vi "A_New Set Point.vi"(0 "T1":dbl, 1 "T2":dbl, 2 "T3":dbl, 3 "T4":dbl, 4 "T5":dbl, 5 "T6":dbl, 6 "T7":dbl, 8 "T8":dbl, 9 "Period":dbl, 10 "T9":dbl, 11 "i":i32, 12 "T10":dbl, 14 "A1":dbl, 15 "A2":dbl, 16 "A3":dbl, 17 "A4":dbl, 18 "A5":dbl, 19 "A6":dbl) -> (13 "y":dbl)   [LabVIEW 2011]
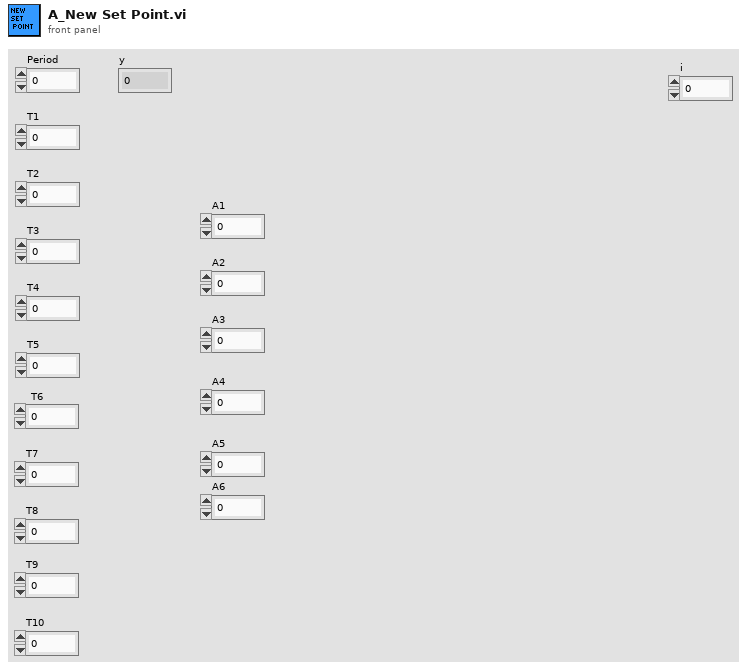
[diagram p1: front panel]
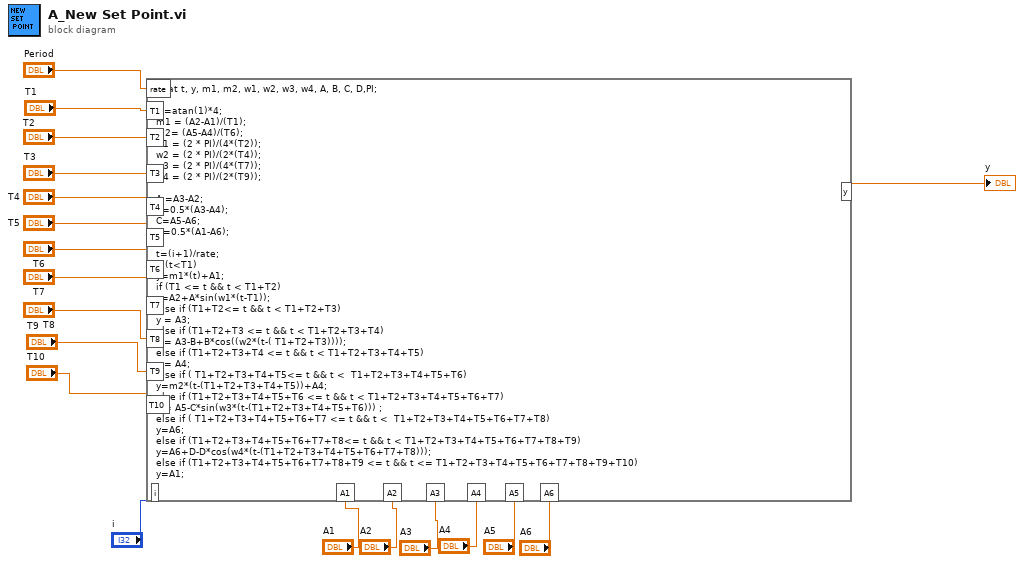
[diagram p0: block diagram]
diagram:
  n1 = formula code="float t, y, m1, m2, w1, w2, w3, w4, A, B, C, D,PI;\n\nPI=atan(1)*4;\nm1 = (A2-A1)/(T1);\nm2= (A5-A4)/(T6);\nw1 = (2 * PI)/(4*(T2));\nw2 = (2 * PI)/(2*(T4));\nw3 = (2 * PI)/(4*(T7));\nw4 = (2 * PI)/(2*(T9));\n\nA =A3-A2;\nB=0.5*(A3-A4);\nC=A5-A6;\nD=0.5*(A1-A6);\n\nt=(i+1)/rate;\nif (t<T1)\ny=m1*(t)+A1;\nif (T1 <= t && t < T1+T2)\ny=A2+A*sin(w1*(t-T1));\nelse if (T1+T2<= t && t < T1+T2+T3)\ny = A3;\nelse if (T1+T2+T3 <= t && t < T1+T2+T3+T4)\ny = A3-B+B*cos((w2*(t-( T1+T2+T3))));\nelse if (T1+T2+T3+T4 <= t && t < T1+T2+T3+T4+T5)\ny = A4;\nelse if ( T1+T2+T3+T4+T5<= t && t <  T1+T2+T3+T4+T5+T6)\ny=m2*(t-(T1+T2+T3+T4+T5))+A4;\nelse if (T1+T2+T3+T4+T5+T6 <= t && t < T1+T2+T3+T4+T5+T6+T7)\ny = A5-C*sin(w3*(t-(T1+T2+T3+T4+T5+T6))) ;\nelse if ( T1+T2+T3+T4+T5+T6+T7 <= t && t <  T1+T2+T3+T4+T5+T6+T7+T8)\ny=A6;\nelse if (T1+T2+T3+T4+T5+T6+T7+T8<= t && t < T1+T2+T3+T4+T5+T6+T7+T8+T9)\ny=A6+D-D*cos(w4*(t-(T1+T2+T3+T4+T5+T6+T7+T8)));\nelse if (T1+T2+T3+T4+T5+T6+T7+T8+T9 <= t && t <= T1+T2+T3+T4+T5+T6+T7+T8+T9+T10)\ny=A1;"("T1"="T1", "T2"="T2", "T3"="T3", "T4"="T4", "T5"="T5", "T6"="T6", "T7"="T7", "T8"="T8", "i"="i", "A1"="A1", "A2"="A2", "A3"="A3", "A4"="A4", "rate"="Period", "T9"="T9", "T10"="T10", "A5"="A5", "A6"="A6") -> ("y"=→"y":dbl)
